vi "SCLN_TCPReadwithSize.vi"(8 "error in (no error)":errorcluster, 9 "timeout ms (600)":i32=600, 11 "connection ID":refnum<k5>) -> (0 "error out":errorcluster, 2 "data out":string, 3 "connection ID out":refnum<k5>)   [LabVIEW 2015]
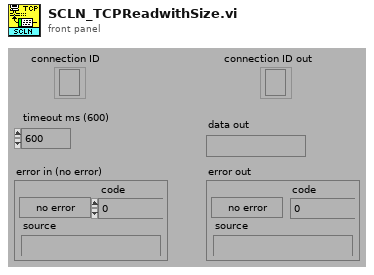
[diagram p1: front panel]
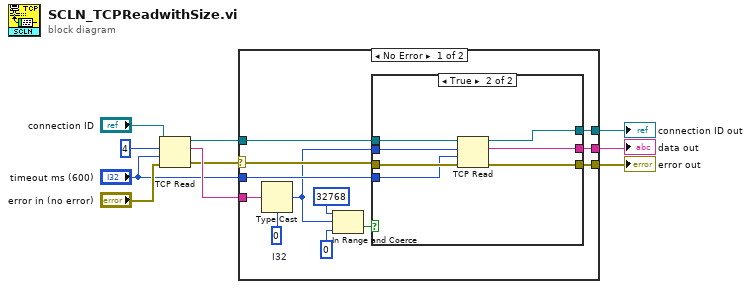
[diagram p0: block diagram]
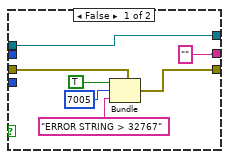
[diagram p2: hidden frame]
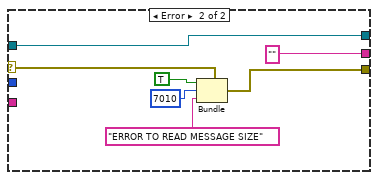
[diagram p3: hidden frame]
diagram:
  n1 = TCP Read(connection ID="connection ID", bytes to read=4, error in (no error)="error in (no error)", 9:"timeout ms (600)") -> (connection ID out=w6:refnum<k5>, data out=w7:string, error out=w1:errorcluster)  [unwired: 1 in]
  n2 = case shown="No Error" w1 {
    selector: w1 -> [w12 w37]
    tunnel: w7 -> [w22 _]
    tunnel: w6 -> [w20 w38]
    tunnel: "timeout ms (600)" -> [w19 _]
    tunnel: [w18 ""] -> w4
    tunnel: [w17 w38] -> w3
    tunnel: [w16 w40] -> w2
    frame No Error {
      w21 = 0  # I32
      n3 = Type Cast(type=w21, x=w22) -> (*(type *) &x=w11:i32)
      n4 = In Range and Coerce(upper limit=32768, x=w11, lower limit=0) -> (In Range?=w13:bool)  [unwired: 1 out]
      n5 = case shown="True" w13 {
        tunnel: w20 -> [w25 w36]
        tunnel: w12 -> [w29 w35]
        tunnel: w19 -> [_ w34]
        tunnel: ["" w33] -> w18
        tunnel: [w25 w32] -> w17
        tunnel: [w24 w31] -> w16
        tunnel: w11 -> [_ w30]
        frame False {
          n6 = Bundle(cluster=w29, "status"=TRUE, "code"=7005, "source"="ERROR STRING > 32767") -> (w24:errorcluster)
        }
        frame True {
          n7 = TCP Read(connection ID=w36, bytes to read=w30, error in (no error)=w35, 9:w34) -> (connection ID out=w32:refnum<k5>, data out=w33:string, error out=w31:errorcluster)  [unwired: 1 in]
        }
      }
    }
    frame Error {
      n8 = Bundle(cluster=w37, "status"=TRUE, "code"=7010, "source"="ERROR TO READ MESSAGE SIZE") -> (w40:errorcluster)
    }
  }
  "data out" <- w4
  "connection ID out" <- w3
  "error out" <- w2
